vi "Query Status Register.vi"(8 "error in (no error)":errorcluster, 11 "36234A in":refnum<class "36234A.lvclass">) -> (0 "error out":errorcluster, 3 "36234A out":refnum<class "36234A.lvclass">)   [LabVIEW 2019, in "36234A.lvlib" / "36234A.lvclass"]
doc: "Child classes must override this VI:\n\nThis VI is the device specific query of the supply's status registers. \nThe return values are: \n\nThe implementation must read status registers and push the status register values to private data for:\nOCP Flag, OVP Flag, Interlock Flag, Output Flag into the private data arrays of the power supply class."
uses:
  Library/36234A.lvclass
  C:/Users/Public/Documents/Development/builds/Instruments/PowerSupply.lvlibp/Library/PowerSupply.lvclass
  builds/Instruments/PowerSupply.lvlibp/Private/Accessors/Read Number of Channels.vi
  builds/Instruments/PowerSupply.lvlibp/Accessors/Write Status Flags.vi
  builds/Instruments/PowerSupply.lvlibp/Library/PowerSupply.lvclass
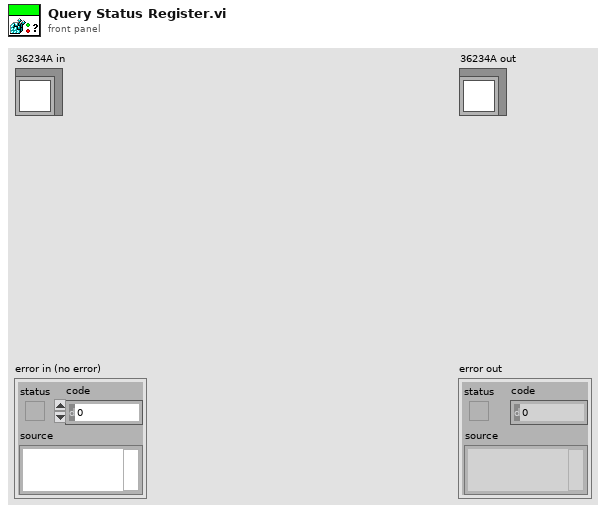
[diagram p1: front panel]
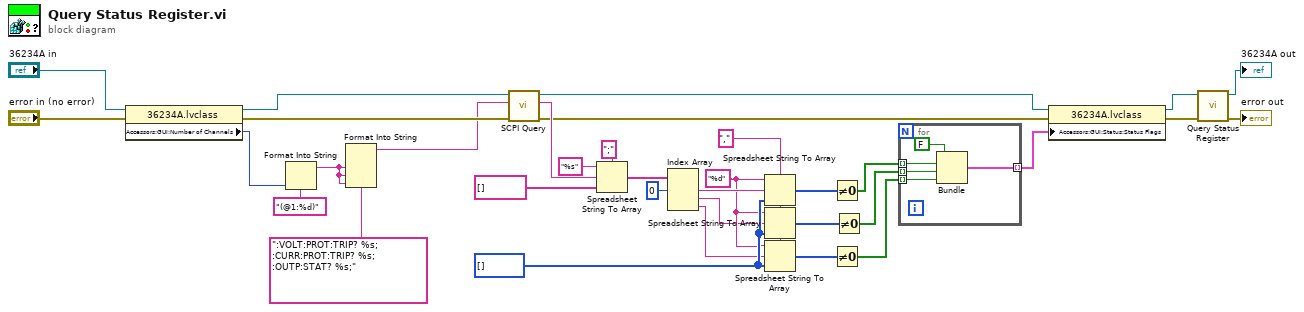
[diagram p0: block diagram]
diagram:
  w13 = i32[] []
  w11 = "," ("delimiter (Tab)")
  w4 = "%d" ("format string")
  n1 = property class="36234A.lvclass"(reference="36234A in", error in="error in (no error)") -> (reference out=w28:refnum<class "36234A.lvclass">, error out=w30:errorcluster, "Accessors:GUI:Number of Channels"=w5:i32)
  n2 = Format Into String(format string="(@1:%d)", w5) -> (resulting string=w17:string)  [unwired: 2 in, 1 out]
  n3 = Format Into String(format string=":VOLT:PROT:TRIP? %s; :CURR:PROT:TRIP? %s; :OUTP:STAT? %s;", w17, w17, w17) -> (resulting string=w22:string)  [unwired: 2 in, 1 out]
  n4 = call "SCPI Query.vi"("error in (no error)"=w30, "SCPI QUERY"=w22, "36234A in"=w28) -> ("error out"=w20:errorcluster, "read buffer"=w25:string, "36234A out"=w21:refnum<class "36234A.lvclass">)  [unwired: 6 in]
  n5 = Spreadsheet String To Array(delimiter (Tab)=";", format string="%s", spreadsheet string=w25, array type (2D Dbl)=string[] []) -> (array=w16:string[])
  n6 = Index Array(array=w16, index #1=0 ("index")) -> (element #1=w14:string, element #2=w3:string, element #3=w2:string)  [unwired: 2 in]
  n7 = Spreadsheet String To Array(delimiter (Tab)=w11, format string=w4, spreadsheet string=w14, array type (2D Dbl)=w13) -> (array=w9:i32[])
  n8 = Spreadsheet String To Array(delimiter (Tab)=w11, format string=w4, spreadsheet string=w3, array type (2D Dbl)=w13) -> (array=w10:i32[])
  n9 = Spreadsheet String To Array(delimiter (Tab)=w11, format string=w4, spreadsheet string=w2, array type (2D Dbl)=w13) -> (array=w12:i32[])
  n10 = Not Equal To 0?(x=w9) -> (x != 0?=w6:bool[])
  n11 = Not Equal To 0?(x=w12) -> (x != 0?=w8:bool[])
  n12 = Not Equal To 0?(x=w10) -> (x != 0?=w7:bool[])
  n13 = for {
    tunnel: [w39] -> w1 mode=indexing
    tunnel: w8 -> [w38] mode=indexing
    tunnel: w7 -> [w37] mode=indexing
    tunnel: w6 -> [w36] mode=indexing
    n14 = Bundle(FALSE, w36, w37, w38) -> (w39:cluster{bool, bool, bool, bool})  [unwired: 1 in]
  }
  n15 = property class="36234A.lvclass"(reference=w21, error in=w20, "Accessors:GUI:Status:Status Flags"=w1) -> (reference out=w19:refnum<class "36234A.lvclass">, error out=w18:errorcluster)
  n16 = call-parent "Query Status Register.vi"("error in (no error)"=w18, "PowerSupply in"=w19) -> ("error out"=→"error out":errorcluster, "PowerSupply out"=→"36234A out":refnum<class "36234A.lvclass">)  [unwired: 8 in]
